vi "PicoLogHRDLExampleStreaming.vi"() -> ()   [LabVIEW 2010]
uses:
  PicohrdlLib/channels.ctl
panel:
  in  "Conversion time":i16(ring) items=["60ms", "100ms", "180ms", "340ms", "660ms"]
  out "Over Range":i16 format="%020b"
  out "error out":errorcluster
  out "handle":i16
  in  "App Buffer size":i32=100
  out "Analog Channels":cluster{i32, dbl, "DataOut":dbl[]}[](graph)
  in  "stop":bool
  out "maxAdc":i32
  in  "Channel Settings":T1={"Ch1"={"1"=TRUE, "Ch 1"=0}, "Ch2"={"2"=TRUE, "Ch 2"=0}, "Ch3"={"3"=FALSE, "Ch 3"=0}, "Ch4"={"4"=FALSE, "Ch 4"=0}, "Ch5"={"5"=FALSE, "Ch 5"=0}, "Ch6"={"6"=FALSE, "Ch 6"=0}, "Ch7"={"7"=FALSE, "Ch 7"=0}, "Ch8"={"8"=FALSE, "Ch 8"=0}, "Ch9"={"9"=FALSE, "Ch 9"=0}, "Ch10"={"10"=FALSE, "Ch 10"=0}, "Ch11"={"11"=FALSE, "Ch 11"=0}, "Ch12"={"12"=FALSE, "Ch 12"=0}, "Ch13"={"13"=FALSE, "Ch 13"=0}, "Ch14"={"14"=FALSE, "Ch 14"=0}, "Ch15"={"15"=FALSE, "Ch 15"=0}, "Ch16"={"16"=FALSE, "Ch 16"=0}, "Ch1/Ch2"={"Single Ended"=TRUE}, "Ch3/Ch4"={"Single Ended"=TRUE}, "Ch5/Ch6"={"Single Ended"=TRUE}, "Ch7/Ch8"={"Single Ended"=TRUE}, "Ch9/Ch10"={"Single Ended"=TRUE}, "Ch11/Ch12"={"Single Ended"=TRUE}, "Ch13/Ch14"={"Single Ended"=TRUE}, "Ch15/Ch16"={"Single Ended"=TRUE}} {"Ch16"."Ch 16" items=["2500mV", "1225mV", "625mV", "313mV", "156mV", "78mV", "39mV"]; "Ch15"."Ch 15" items=["2500mV", "1225mV", "625mV", "313mV", "156mV", "78mV", "39mV"]; "Ch14"."Ch 14" items=["2500mV", "1225mV", "625mV", "313mV", "156mV", "78mV", "39mV"]; "Ch13"."Ch 13" items=["2500mV", "1225mV", "625mV", "313mV", "156mV", "78mV", "39mV"]; "Ch12"."Ch 12" items=["2500mV", "1225mV", "625mV", "313mV", "156mV", "78mV", "39mV"]; "Ch11"."Ch 11" items=["2500mV", "1225mV", "625mV", "313mV", "156mV", "78mV", "39mV"]; "Ch10"."Ch 10" items=["2500mV", "1225mV", "625mV", "313mV", "156mV", "78mV", "39mV"]; "Ch9"."Ch 9" items=["2500mV", "1225mV", "625mV", "313mV", "156mV", "78mV", "39mV"]; "Ch8"."Ch 8" items=["2500mV", "1225mV", "625mV", "313mV", "156mV", "78mV", "39mV"]; "Ch7"."Ch 7" items=["2500mV", "1225mV", "625mV", "313mV", "156mV", "78mV", "39mV"]; "Ch6"."Ch 6" items=["2500mV", "1225mV", "625mV", "313mV", "156mV", "78mV", "39mV"]; "Ch5"."Ch 5" items=["2500mV", "1225mV", "625mV", "313mV", "156mV", "78mV", "39mV"]; "Ch4"."Ch 4" items=["2500mV", "1225mV", "625mV", "313mV", "156mV", "78mV", "39mV"]; "Ch3"."Ch 3" items=["2500mV", "1225mV", "625mV", "313mV", "156mV", "78mV", "39mV"]; "Ch2"."Ch 2" items=["2500mV", "1225mV", "625mV", "313mV", "156mV", "78mV", "39mV"]; "Ch1"."Ch 1" items=["2500mV", "1225mV", "625mV", "313mV", "156mV", "78mV", "39mV"]}
  out "sampleInterval_ms":i32
  in  "Mains Frequency":i16(ring) items=["50 Hz", "60 Hz"]
  out "noOfChannels":i16
  out "Channel Enable Array":i32[](array[numeric])=[0, 1, 1, 0, 0, 0, 0, 0, 0, 0, 0, 0, 0, 0, 0, 0]
  in  "error in (no error)":errorcluster
  out "Unit Info":T2
  # "NOTES-\nNumber of channels-\nADC-20: 1 to 8\nADC-24: 1 to 16\n\nIf the channel pair\n(Ch1 & Ch2 for example) is set to differential mode then the odd number channel controls are used. \n\nRange Voltage range Availability\n (0)    ±2500 mV        ADC-20 and ADC-24\n (1)    ±1250 mV        ADC-20 and ADC-24\n (2)    ±625 mV          ADC-24 only\n (3)    ±312.5 mV       ADC-24 only\n (4)    ±156.25 mV     ADC-24 only\n (5)    ±78.125 mV     ADC-24 only\n (6)    ±39.0625 mV   ADC-24 only"
  # "Diff."
  # "Diff."
  # "Diff."
  # "Diff."
  # "Diff."
  # "Diff."
  # "Diff."
  # "Diff."
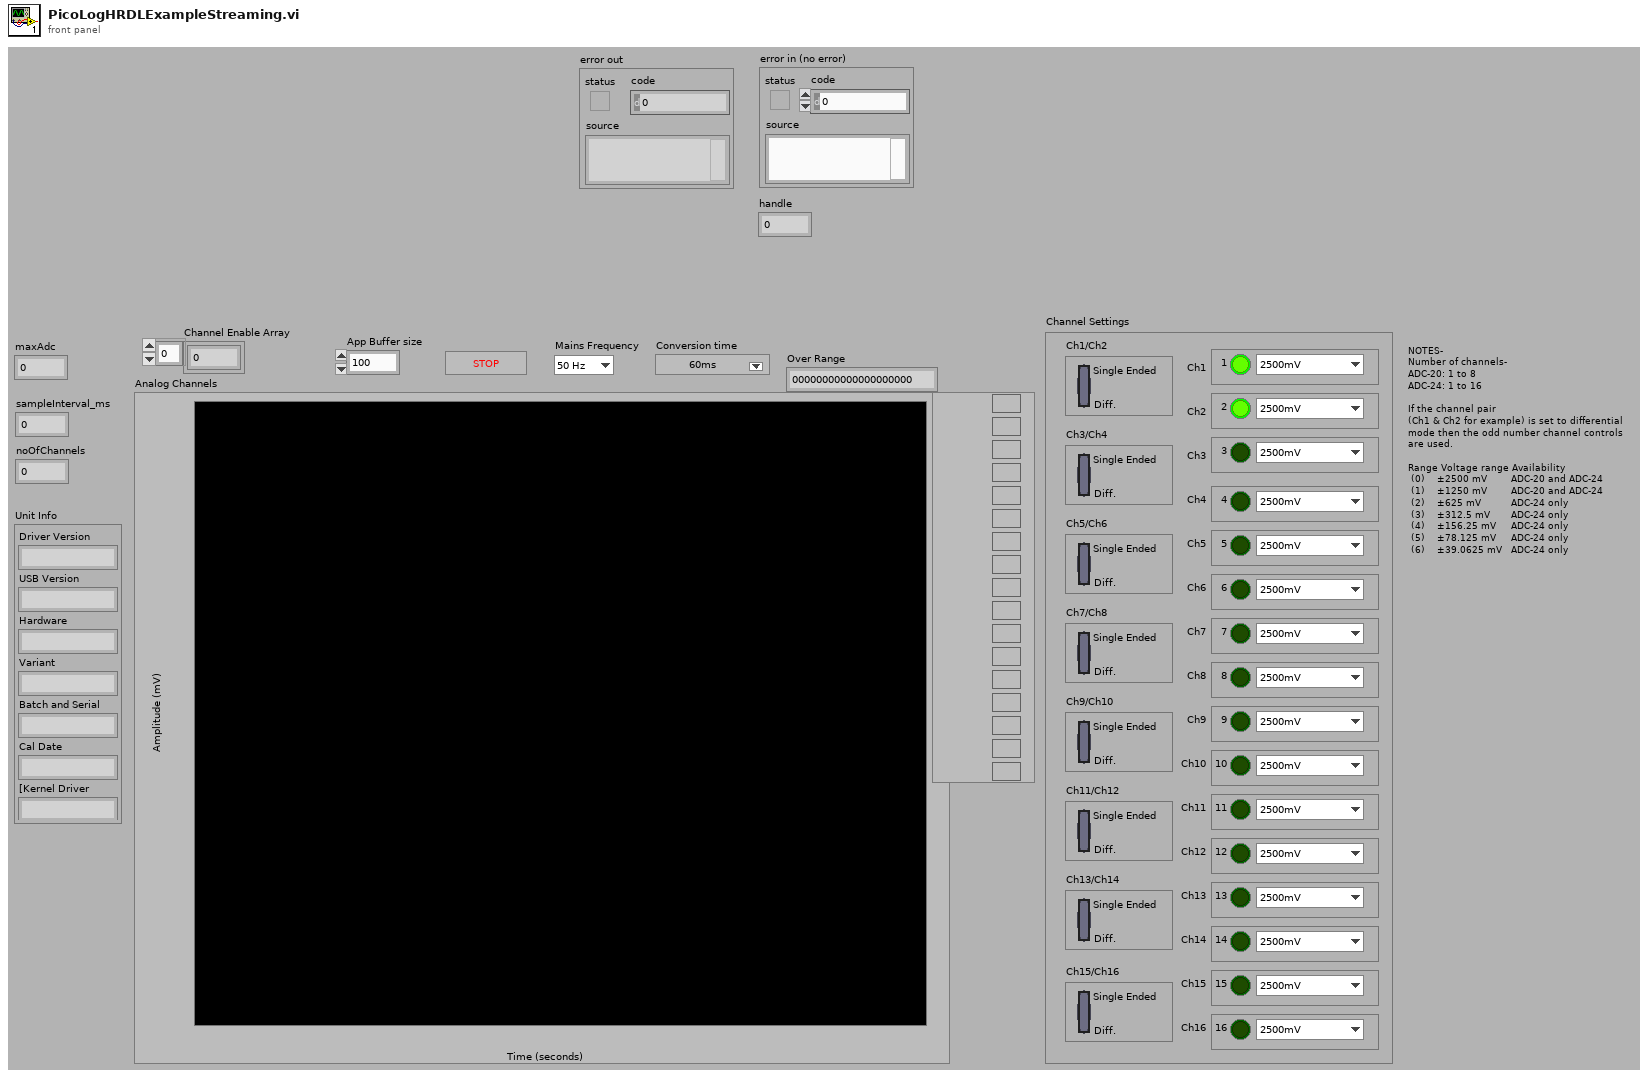
[diagram p1: front panel]
types:
  T1 = typedef "channels.ctl" = cluster{"Ch1":cluster{"1":bool, "Ch 1":i16}, "Ch2":cluster{"2":bool, "Ch 2":i16}, "Ch3":cluster{"3":bool, "Ch 3":i16}, "Ch4":cluster{"4":bool, "Ch 4":i16}, "Ch5":cluster{"5":bool, "Ch 5":i16}, "Ch6":cluster{"6":bool, "Ch 6":i16}, "Ch7":cluster{"7":bool, "Ch 7":i16}, "Ch8":cluster{"8":bool, "Ch 8":i16}, "Ch9":cluster{"9":bool, "Ch 9":i16}, "Ch10":cluster{"10":bool, "Ch 10":i16}, "Ch11":cluster{"11":bool, "Ch 11":i16}, "Ch12":cluster{"12":bool, "Ch 12":i16}, "Ch13":cluster{"13":bool, "Ch 13":i16}, "Ch14":cluster{"14":bool, "Ch 14":i16}, "Ch15":cluster{"15":bool, "Ch 15":i16}, "Ch16":cluster{"16":bool, "Ch 16":i16}, "Ch1/Ch2":cluster{"Single Ended":bool}, "Ch3/Ch4":cluster{"Single Ended":bool}, "Ch5/Ch6":cluster{"Single Ended":bool}, "Ch7/Ch8":cluster{"Single Ended":bool}, "Ch9/Ch10":cluster{"Single Ended":bool}, "Ch11/Ch12":cluster{"Single Ended":bool}, "Ch13/Ch14":cluster{"Single Ended":bool}, "Ch15/Ch16":cluster{"Single Ended":bool}}
  T2 = cluster{"Driver Version":string, "USB Version":string, "Hardware":string, "Variant":string, "Batch and Serial":string, "Cal Date":string, "[Kernel Driver":string, "[7]":string, "[8]":string, "[9]":string, "[10]":string, "[11]":string, "[12]":string, "[13]":string, "[14]":string}
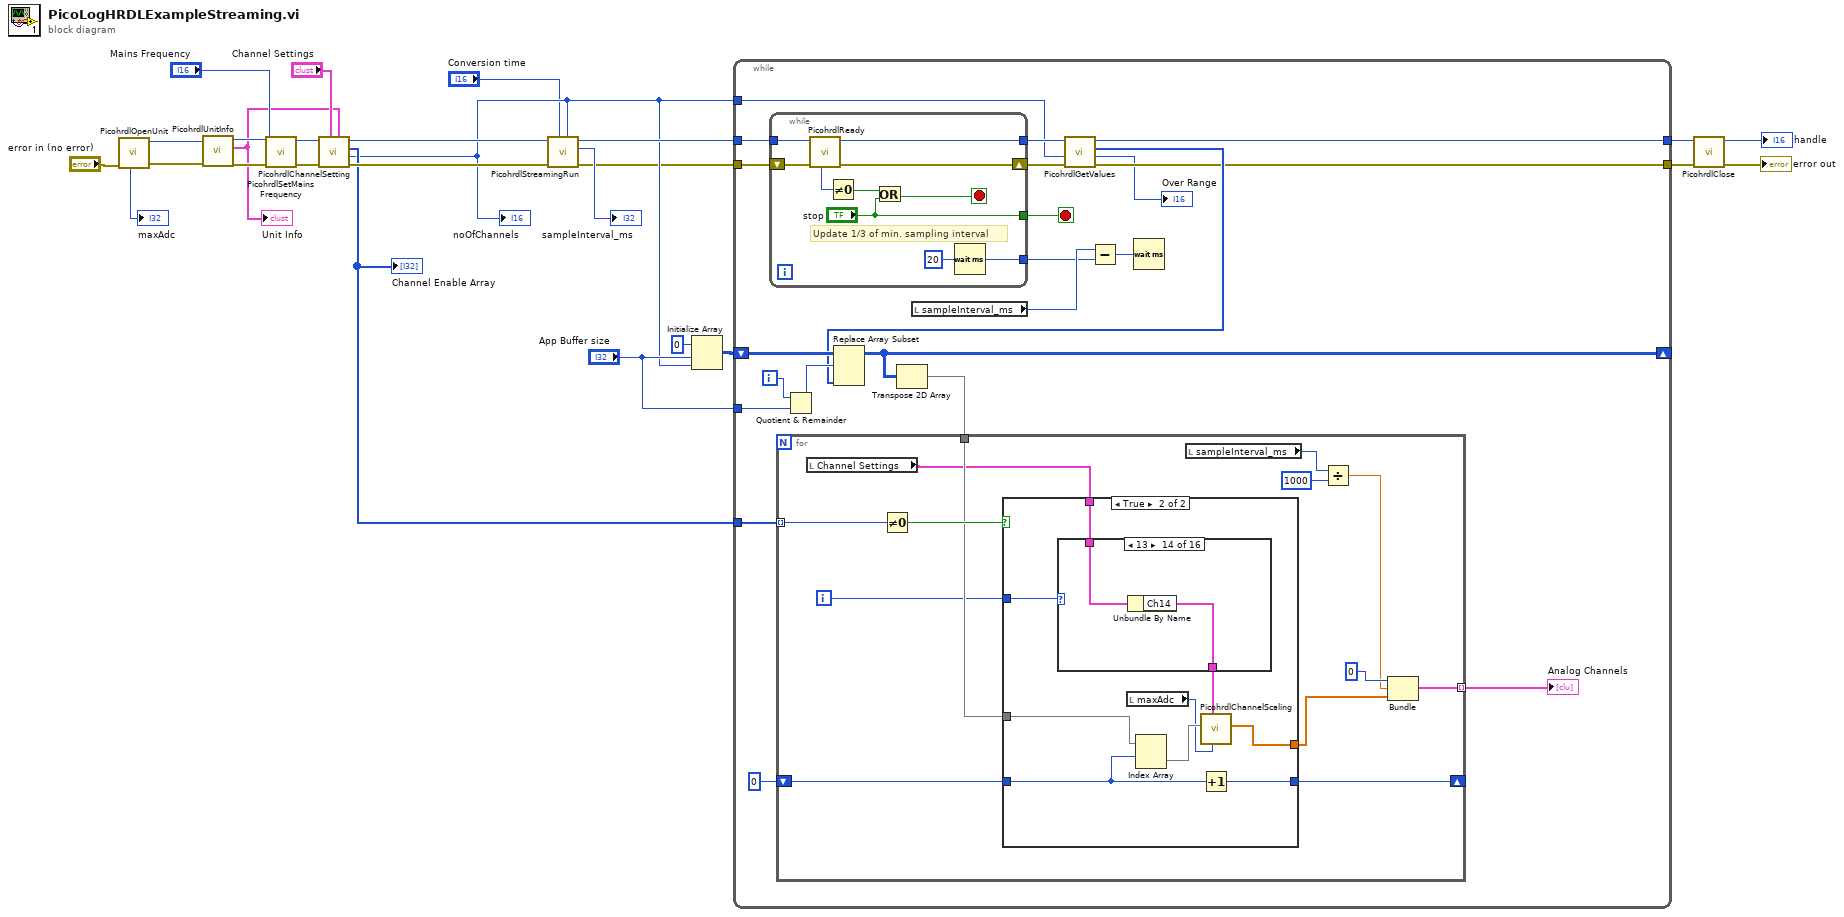
[diagram p0: block diagram]
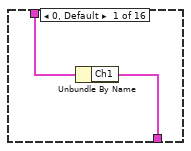
[diagram p3: hidden frame]
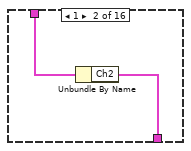
[diagram p4: hidden frame]
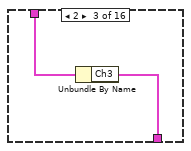
[diagram p5: hidden frame]
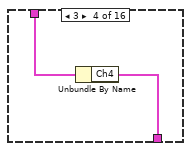
[diagram p6: hidden frame]
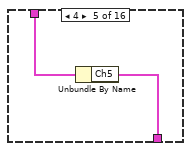
[diagram p7: hidden frame]
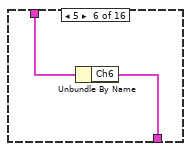
[diagram p8: hidden frame]
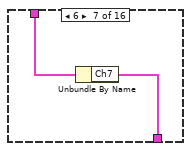
[diagram p9: hidden frame]
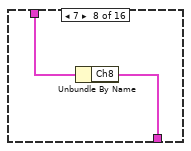
[diagram p10: hidden frame]
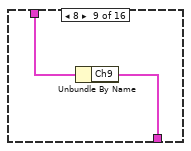
[diagram p11: hidden frame]
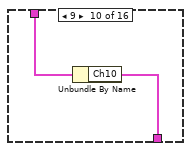
[diagram p12: hidden frame]
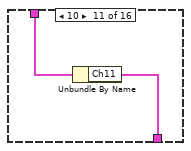
[diagram p13: hidden frame]
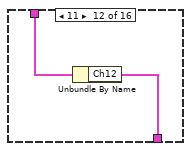
[diagram p14: hidden frame]
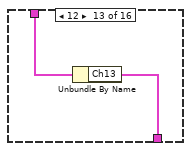
[diagram p15: hidden frame]
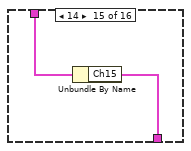
[diagram p16: hidden frame]
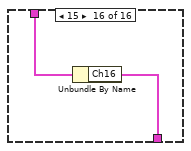
[diagram p17: hidden frame]
diagram:
  n1 = call "PicohrdlOpenUnit.vi"("error in (no error)"="error in (no error)") -> ("error out"=w11:errorcluster, "Handle out"=w6:i16, "maxAdc"=→"maxAdc":i32)  [unwired: 7 in, 1 out]
  n2 = call "PicohrdlUnitInfo.vi"("error in (no error)"=w11, "handle in"=w6) -> ("error out"=w10:errorcluster, "Unit Info"=w7:T2, "handle out"=w9:i16)  [unwired: 7 in]
  "Unit Info" <- w7
  n3 = call "PicohrdlSetMainsFrequency.vi"("error in (no error)"=w10, "Mains Frequency"="Mains Frequency", "Handle in"=w9) -> ("error out"=w23:errorcluster, "Handle out"=w24:i16)  [unwired: 7 in]
  n4 = call "PicohrdlChannelSetting.vi"("Unit Info"=w7, "Channel Settings"="Channel Settings", "error in (no error)"=w23, "Handle In"=w24) -> ("error out"=w21:errorcluster, "noOfChannels"=w13:i16, "Channel Enable Array"=w18:i32[], "Handle out"=w20:i16)  [unwired: 4 in]
  "Channel Enable Array" <- w18
  "noOfChannels" <- w13
  n5 = call "PicohrdlStreamingRun.vi"("noOfChannels"=w13, "conversionTime"="Conversion time", "error in (no error)"=w21, "Handle in"=w20) -> ("error out"=w8:errorcluster, "sampleInterval_ms"=→"sampleInterval_ms":i32, "Handle out"=w19:i16)  [unwired: 5 in]
  n6 = Initialize Array(0 ("element"), "App Buffer size", w13) -> (w15:i32[][])
  n7 = while {
    tunnel: w19 -> [w48]
    tunnel: [w42] -> w25
    tunnel: w13 -> [w39]
    tunnel: w18 -> [w41]
    shift-right: [w36] -> _
    shift-left: w15 -> [w40]
    tunnel: "App Buffer size" -> [w33]
    tunnel: [w30] -> w2
    tunnel: w8 -> [w28]
    i -> [w34]
    stop <- w47 stop-if-true
    n8 = while {
      tunnel: w48 -> [w105]
      tunnel: [w111] -> w43
      tunnel: ["stop"] -> w47
      tunnel: [w110] -> w44
      shift-right: [w107] -> w29
      shift-left: w28 -> [w106]
      stop <- w104 stop-if-true
      w110 = u32 20 ("milliseconds to wait")
      # "Update 1/3 of min. sampling interval"
      n9 = call "PicohrdlReady.vi"("error in (no error)"=w106, "handle in"=w105) -> ("error out"=w107:errorcluster, "handle out"=w111:i16, "ready"=w108:i16)  [unwired: 7 in]
      n10 = Not Equal To 0?(x=w108) -> (x != 0?=w112:bool)
      n11 = Or(x=w112, y="stop") -> (x .or. y?=w104:bool)
      n12 = Wait (ms)(milliseconds to wait=w110) -> ()  [unwired: 1 out]
    }
    n13 = Quotient & Remainder(x=w34, y=w33) -> (x-y*floor(x/y)=w35:i32)  [unwired: 1 out]
    n14 = local read "sampleInterval_ms"() -> (w46:i32)
    n15 = call "PicohrdlGetValues.vi"("error in (no error)"=w29, "noOfChannels"=w39, "Handle in"=w43) -> ("error out"=w30:errorcluster, "Overflow"=→"Over Range":i16, "temp_buffer"=w32:i32[], "Handle out"=w42:i16)  [unwired: 5 in]
    n16 = Replace Array Subset(array=w40, new element=w32, index (row)=w35) -> (w36:i32[][])  [unwired: 1 in]
    n17 = Transpose 2D Array(2D array=w36) -> (transposed array=w37:i32[][])
    n18 = for {
      tunnel: w41 -> [w58] mode=indexing
      tunnel: w37 -> [w59]
      shift-right: [w57] -> _
      shift-left: i16 0 ("noOfChannels") -> [w60]
      tunnel: [w52] -> w31 mode=indexing
      i -> [w55]
      n19 = local read "Channel Settings"() -> (w56:T1)
      n20 = Not Equal To 0?(x=w58) -> (x != 0?=w61:bool)
      n21 = case shown="True" w61 {
        tunnel: [_ w69] -> w54
        tunnel: w59 -> [_ w71]
        tunnel: w60 -> [w62 w64]
        tunnel: [w62 w63] -> w57
        tunnel: w56 -> [_ w67]
        tunnel: w55 -> [_ w65]
        frame False {
        }
        frame True {
          n22 = case shown="13" w65 {
            tunnel: w67 -> [w73 w75 w77 w79 w81 w83 w85 w87 w89 w91 w93 w95 w97 w99 w101 w103]
            tunnel: [w72 w74 w76 w78 w80 w82 w84 w86 w88 w90 w92 w94 w96 w98 w100 w102] -> w66
            frame 0, Default {
              n23 = Unbundle By Name(w73) -> ("Ch1"=w72:cluster{"1":bool, "Ch 1":i16})
            }
            frame 1 {
              n24 = Unbundle By Name(w75) -> ("Ch2"=w74:cluster{"2":bool, "Ch 2":i16})
            }
            frame 2 {
              n25 = Unbundle By Name(w77) -> ("Ch3"=w76:cluster{"3":bool, "Ch 3":i16})
            }
            frame 3 {
              n26 = Unbundle By Name(w79) -> ("Ch4"=w78:cluster{"4":bool, "Ch 4":i16})
            }
            frame 4 {
              n27 = Unbundle By Name(w81) -> ("Ch5"=w80:cluster{"5":bool, "Ch 5":i16})
            }
            frame 5 {
              n28 = Unbundle By Name(w83) -> ("Ch6"=w82:cluster{"6":bool, "Ch 6":i16})
            }
            frame 6 {
              n29 = Unbundle By Name(w85) -> ("Ch7"=w84:cluster{"7":bool, "Ch 7":i16})
            }
            frame 7 {
              n30 = Unbundle By Name(w87) -> ("Ch8"=w86:cluster{"8":bool, "Ch 8":i16})
            }
            frame 8 {
              n31 = Unbundle By Name(w89) -> ("Ch9"=w88:cluster{"9":bool, "Ch 9":i16})
            }
            frame 9 {
              n32 = Unbundle By Name(w91) -> ("Ch10"=w90:cluster{"10":bool, "Ch 10":i16})
            }
            frame 10 {
              n33 = Unbundle By Name(w93) -> ("Ch11"=w92:cluster{"11":bool, "Ch 11":i16})
            }
            frame 11 {
              n34 = Unbundle By Name(w95) -> ("Ch12"=w94:cluster{"12":bool, "Ch 12":i16})
            }
            frame 12 {
              n35 = Unbundle By Name(w97) -> ("Ch13"=w96:cluster{"13":bool, "Ch 13":i16})
            }
            frame 13 {
              n36 = Unbundle By Name(w99) -> ("Ch14"=w98:cluster{"14":bool, "Ch 14":i16})
            }
            frame 14 {
              n37 = Unbundle By Name(w101) -> ("Ch15"=w100:cluster{"15":bool, "Ch 15":i16})
            }
            frame 15 {
              n38 = Unbundle By Name(w103) -> ("Ch16"=w102:cluster{"16":bool, "Ch 16":i16})
            }
          }
          n39 = local read "maxAdc"() -> (w68:i32)
          n40 = Index Array(array=w71, index (row)=w64) -> (element=w70:i32[])  [unwired: 1 in]
          n41 = call "PicohrdlChannelScaling.vi"("Max_adc"=w68, "Channel N"=w66, "DataIn"=w70) -> ("DataOut"=w69:dbl[])  [unwired: 8 in]
          n42 = Increment(x=w64) -> (x+1=w63:i16)
        }
      }
      n43 = local read "sampleInterval_ms"() -> (w51:i32)
      n44 = Divide(x=w51, y=1000) -> (x/y=w49:dbl)
      n45 = Bundle(0, w49, "DataOut"=w54) -> (w52:cluster{i32, dbl, "DataOut":dbl[]})  [unwired: 1 in]
    }
    "Analog Channels" <- w31
    n46 = Subtract(x=w46, y=w44) -> (x-y=w45:u32)
    n47 = Wait (ms)(milliseconds to wait=w45) -> ()  [unwired: 1 out]
  }
  n48 = call "PicohrdlClose.vi"("error in (no error)"=w2, "Handle in"=w25) -> ("error out"=→"error out":errorcluster, "handle"=→"handle":i16)  [unwired: 8 in]
